vi "Create One Frame Script.vi"(8 "error in (no error)":errorcluster, 10 "Config String":string, 11 "SPI 3W Pattern Creator in":refnum<class "SPI 3W Pattern Creator.lvclass">) -> (0 "error out":errorcluster, 1 "Pattern Name out":string, 2 "Script out":string, 3 "SPI 3W Pattern Creator out":refnum<class "SPI 3W Pattern Creator.lvclass">)   [LabVIEW 2018, in "SPI 3W Pattern Creator.lvlib" / "SPI 3W Pattern Creator.lvclass"]
uses:
  SPI 3W Pattern Creator.lvclass
  C:/P4 Workspace/PC Client/Solutions/5g_eap/trunk/1.0/HiSi5GmmWave/Pattern_Gen_Tool/Plugins/Protocols/SPI Root Pattern Creator.lvlibp/Plugins/SouceCode/SPI_Pattern Creator/SPI Root/SPI Root Pattern Creator.lvclass
  Protocols/SPI Root Pattern Creator.lvlibp/Plugins/SouceCode/SPI_Pattern Creator/SPI Root/Read R_W_.vi
  Protocols/SPI Root Pattern Creator.lvlibp/Plugins/SouceCode/SPI_Pattern Creator/SPI Root/Read FRM Data.vi
  Protocols/SPI Root Pattern Creator.lvlibp/Plugins/SouceCode/SPI_Pattern Creator/SPI Root/Read Pattern Name.vi
  Protocols/SPI Root Pattern Creator.lvlibp/Plugins/SouceCode/SPI_Pattern Creator/SPI Root/SPI Root Pattern Creator.lvclass
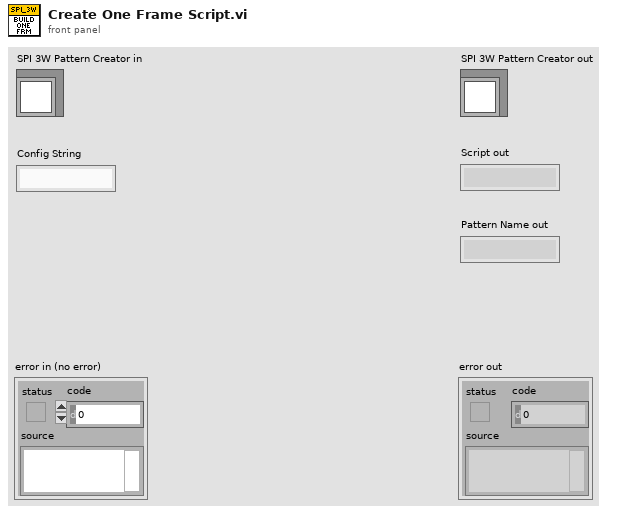
[diagram p1: front panel]
types:
  T1 = typedef "SPI Root Pattern Creator.lvlibp/RW Options.ctl" = enum16{"Read", "Write", "R/W"}
  T2 = typedef "SPI Root Pattern Creator.lvlibp/Frame Data - SPI_3W.ctl" = cluster{"Pattern Name":string, "Data":u16, "Addr":u16, "OpCode":string[], "R/W?":T1}
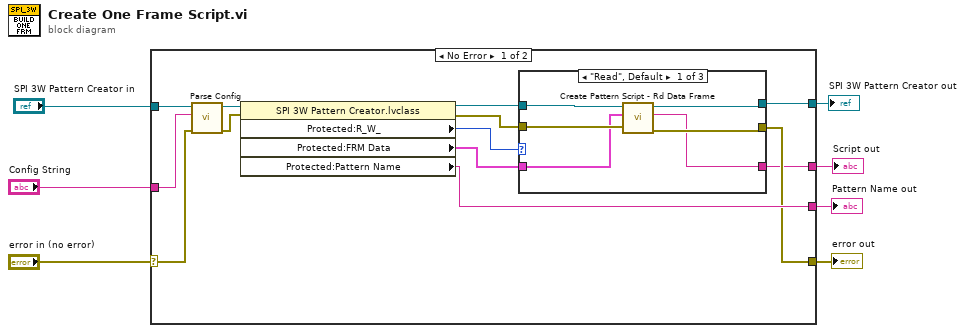
[diagram p0: block diagram]
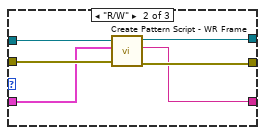
[diagram p2: hidden frame]
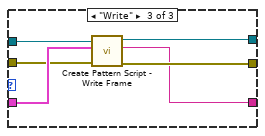
[diagram p3: hidden frame]
diagram:
  n1 = case shown="No Error" "error in (no error)" {
    selector: "error in (no error)" -> [w10 w40]
    tunnel: "SPI 3W Pattern Creator in" -> [w12 w39]
    tunnel: "Config String" -> [w11 _]
    tunnel: [w16 w39] -> w4
    tunnel: [w15 _] -> w3
    tunnel: [w14 w40] -> w2
    tunnel: [w13 _] -> w1
    frame No Error {
      n2 = call "Parse Config.vi"("error in (no error)"=w10, "Config String"=w11, "SPI Root Pattern Creator in"=w12) -> ("error out"=w8:errorcluster, "SPI Root Pattern Creator out"=w9:refnum<class "SPI 3W Pattern Creator.lvclass">)  [unwired: 7 in]
      n3 = property class="SPI 3W Pattern Creator.lvclass"(reference=w9, error in=w8) -> (reference out=w18:refnum<class "SPI 3W Pattern Creator.lvclass">, error out=w19:errorcluster, "Protected:R_W_"=w20:T1, "Protected:FRM Data"=w17:T2, "Protected:Pattern Name"=w15:string)
      n4 = case shown="\"Read\", Default" w20 {
        tunnel: w19 -> [w24 w30 w36]
        tunnel: w18 -> [w26 w32 w38]
        tunnel: w17 -> [w21 w27 w37]
        tunnel: [w25 w31 w35] -> w16
        tunnel: [w23 w29 w34] -> w14
        tunnel: [w22 w28 w33] -> w13
        frame "Read", Default {
          n5 = call-dynamic "Create Pattern Script - Rd Data Frame.vi"("error in (no error)"=w24, "FRM Data"=w21, "SPI 3W Pattern Creator in"=w26) -> ("error out"=w23:errorcluster, "String"=w22:string, "SPI 3W Pattern Creator out"=w25:refnum<class "SPI 3W Pattern Creator.lvclass">)  [unwired: 6 in]
        }
        frame "R/W" {
          n6 = call-dynamic "Create Pattern Script - WR Frame.vi"("error in (no error)"=w30, "FRM Data"=w27, "SPI 3W Pattern Creator in"=w32) -> ("error out"=w29:errorcluster, "String"=w28:string, "SPI 3W Pattern Creator out"=w31:refnum<class "SPI 3W Pattern Creator.lvclass">)  [unwired: 6 in]
        }
        frame "Write" {
          n7 = call-dynamic "Create Pattern Script - Write Frame.vi"("error in (no error)"=w36, "FRM Data"=w37, "SPI 3W Pattern Creator in"=w38) -> ("error out"=w34:errorcluster, "String"=w33:string, "SPI 3W Pattern Creator out"=w35:refnum<class "SPI 3W Pattern Creator.lvclass">)  [unwired: 6 in]
        }
      }
    }
    frame Error {
    }
  }
  "error out" <- w2
  "SPI 3W Pattern Creator out" <- w4
  "Script out" <- w1
  "Pattern Name out" <- w3
